vi "Main_verRockwell.vi"() -> ()   [LabVIEW 2014]
uses:
  <vilib>/ethernetip/ethernetip.llb/EthernetIP Tag Write BOOL.vi
  <vilib>/ethernetip/ethernetip.llb/EthernetIP Tag Write REAL.vi
  <vilib>/ethernetip/ethernetip.lvlib
  <vilib>/vision/driver/NI_Vision_Acquisition_Software.lvlib
panel:
  out "B":bool caption="Running"
  out "G":bool caption="Running"
  out "R":bool caption="Running"
  in  "Motion Speed":u32[](array[knob])=[80] scale=0.0..500.0
  in  "Linear Actuator Limit":u32(slide)=70 scale=0.0..100.0
  out "Linear Actuator Position Graph":dbl[][](graph)
  in  "Next Motion Delay":u32(slide)=200 scale=0.0..900.0
  in  "R Position":u32[](array[knob])=[35] scale=0.0..100.0
  in  "L Position":u32[](array[knob])=[40] scale=0.0..100.0
  in  "PORT":u16=50
  in  "IP":string="127.0.0.1"
  in  "Running Game":string="DiRT 3"
  out "Loop Count":i32=6322
  in  "Error RESET":bool
  in  "Simtools ON":bool
  in  "Motor Start":bool
  in  "Motor Reset":bool
  in  "STOP":bool
  in  "LED":bool
  in  "Axis":bool
  out "Running":bool
  in  "Error In":errorcluster
  out "Error Out":errorcluster
  out "R Position":dbl
  out "L Position":dbl
  out "Axis":string="L127R127C127"
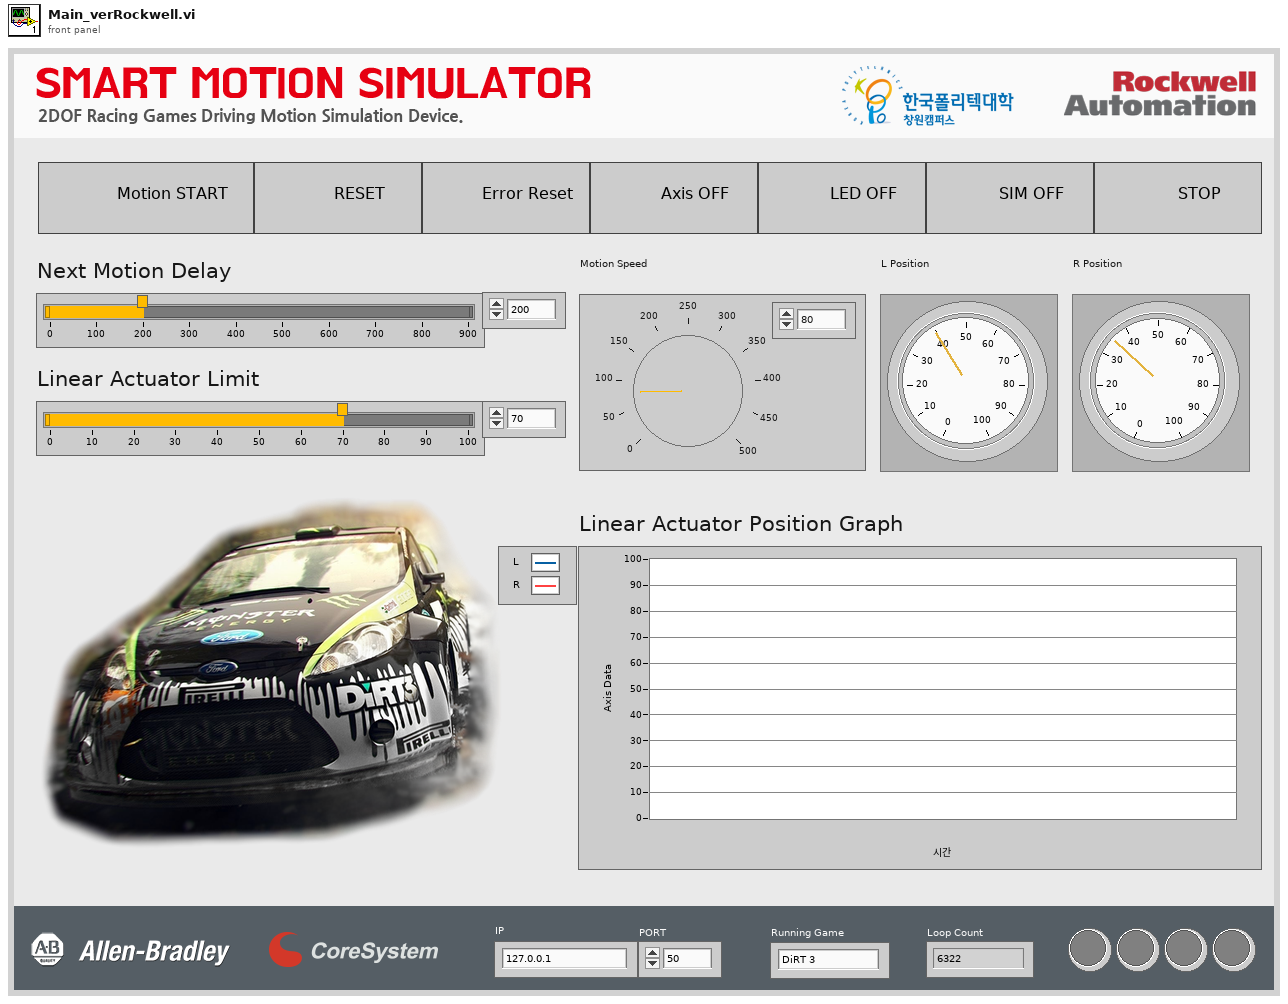
[diagram p1: front panel]
types:
  T1 = typedef "IMAQdx.ctl" = refnum<k21>
  T2 = typedef "IMAQ Image.ctl" = refnum<image>
  T3 = typedef "ethernetip.lvlib/ethernetip.ctl" = refnum<k21>
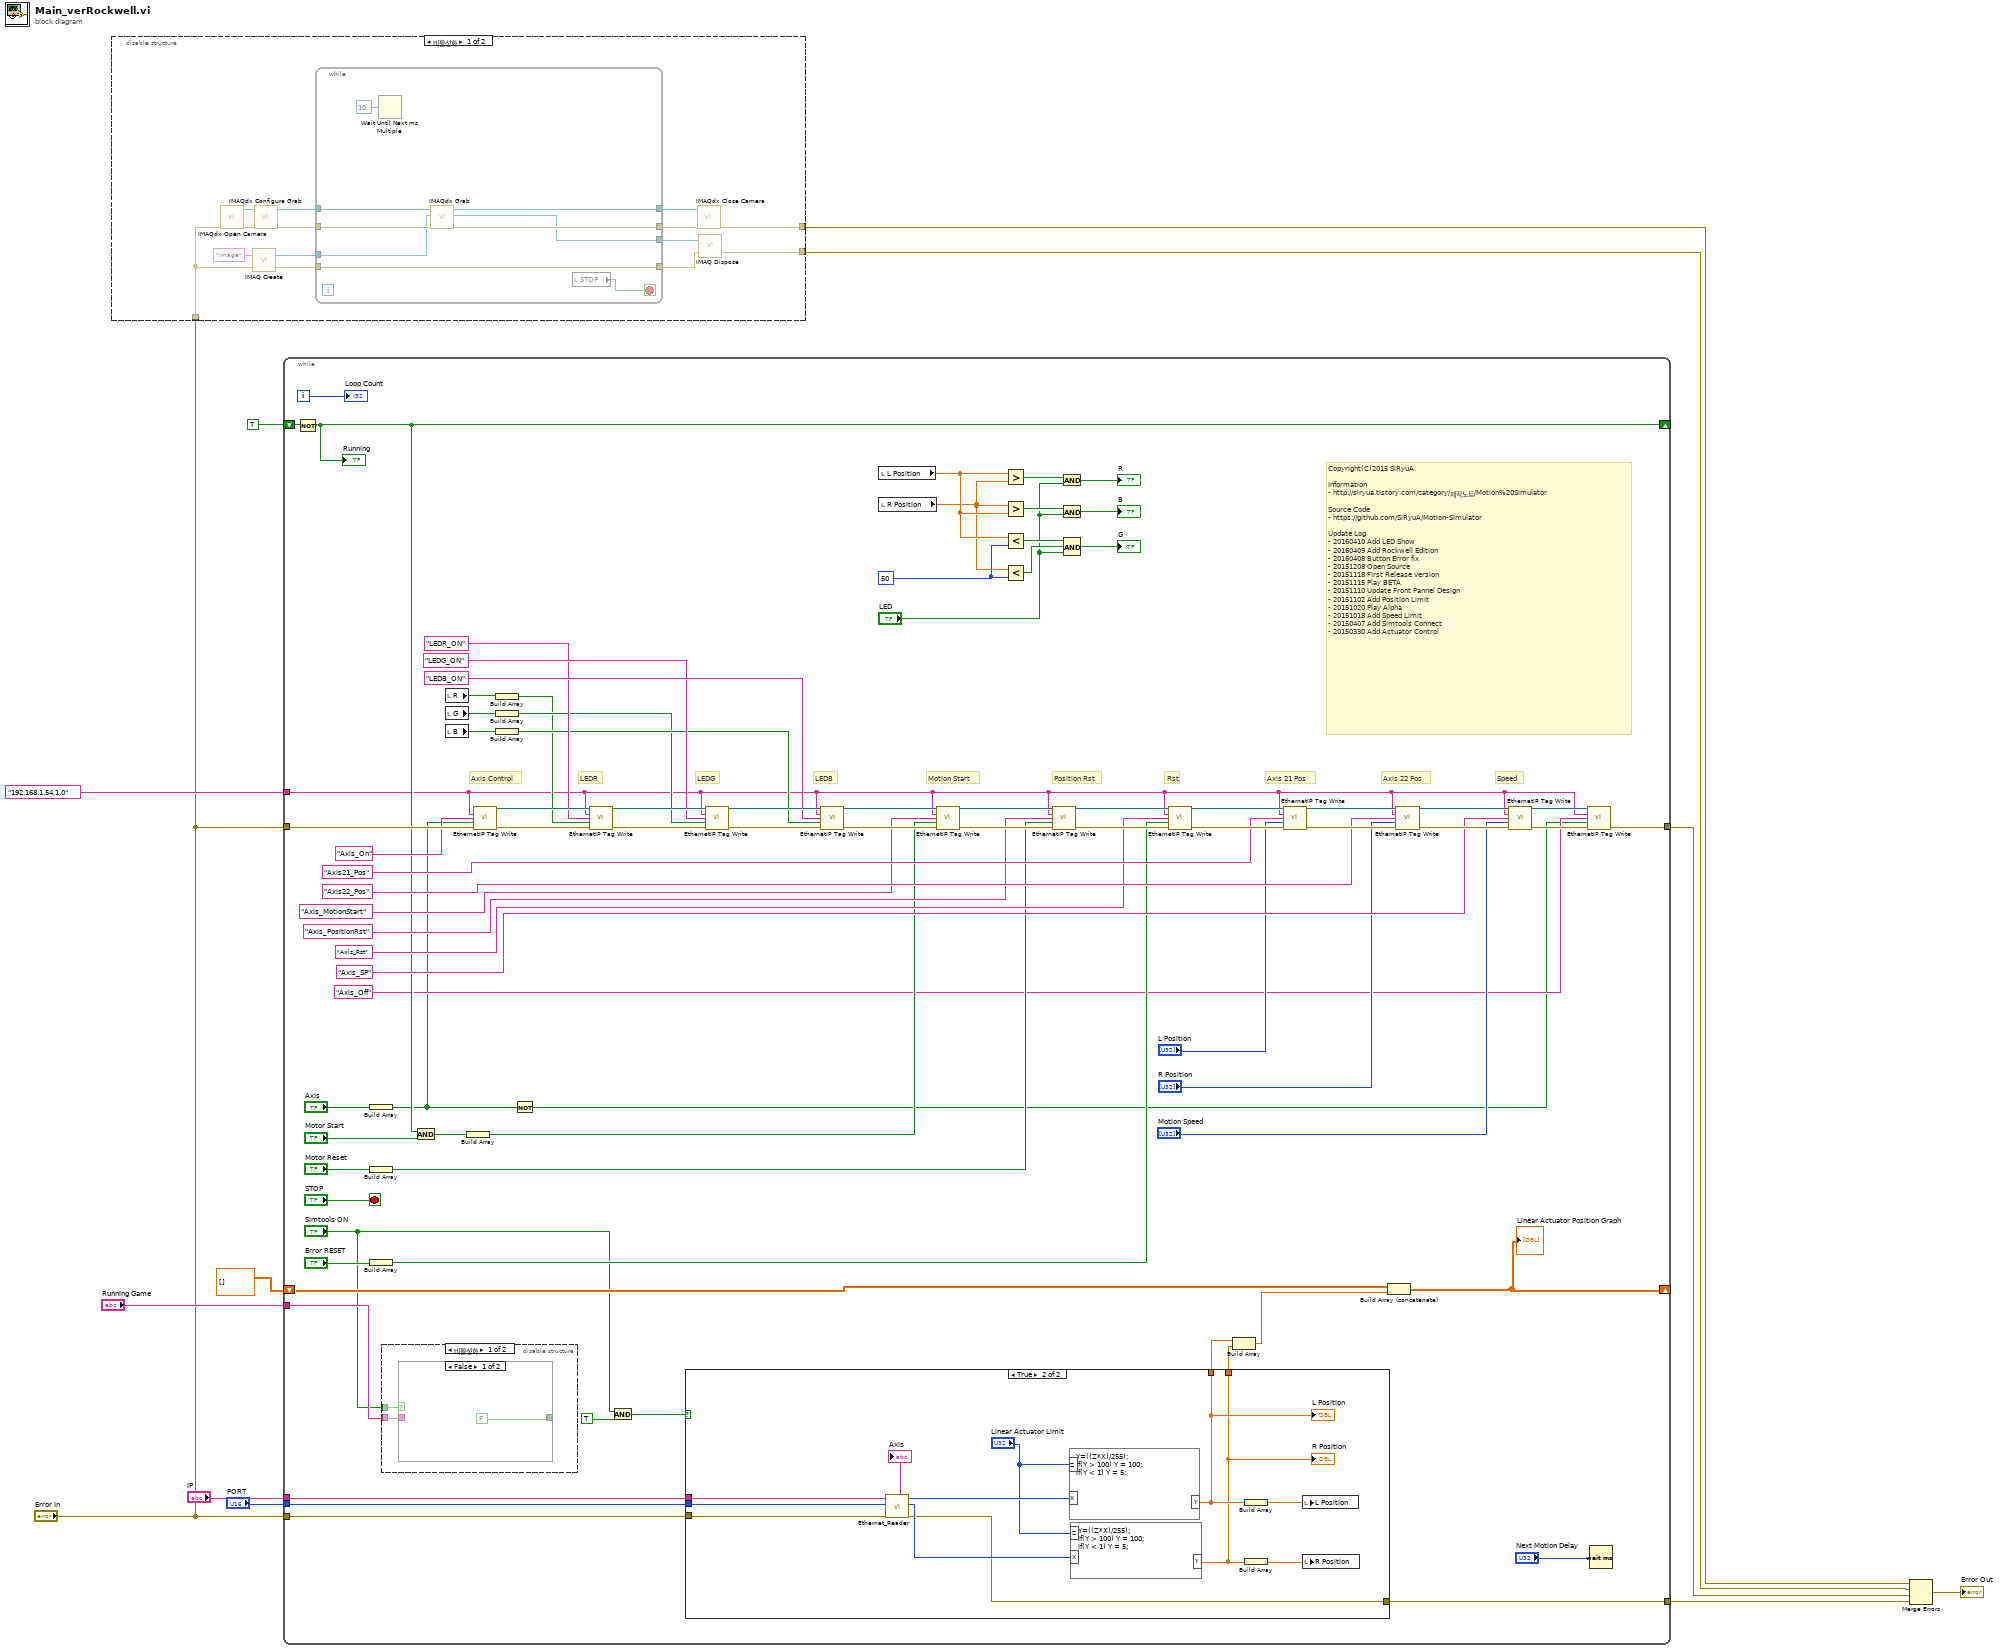
[diagram p0: block diagram]
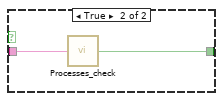
[diagram p3: hidden frame]
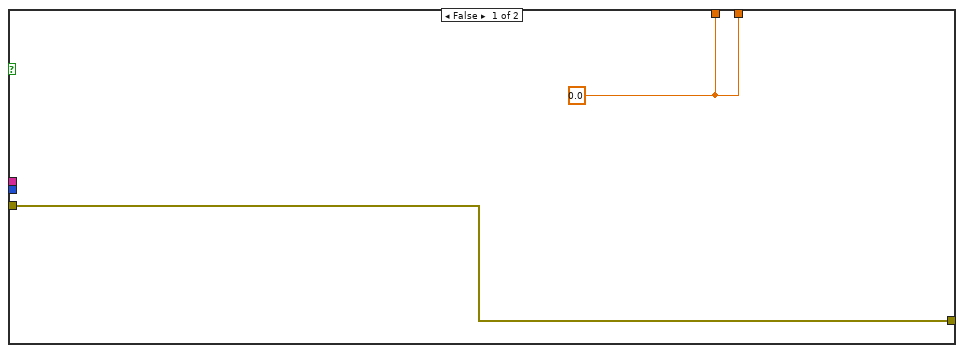
[diagram p5: hidden frame]
diagram:
  n1 = disable-structure shown="비활성화" {
    disable-tunnel: [w23 _] -> w6
    disable-tunnel: [w22 _] -> w5
    disable-tunnel: "Error In" -> [w21 _]
    frame Disabled {
      n2 = call <vilib>:"IMAQdx Open Camera.vi"("error in"=w21) -> ("error out"=w25:errorcluster, "Session Out"=w26:T1, "Session In"=w27:T1)  [unwired: 8 in]
      n3 = call "IMAQ Create"("Image Name"="Image", "error in (no error)"=w21) -> ("New Image"=w16:T2, "error out"=w14:errorcluster)  [unwired: 3 in]
      n4 = call <vilib>:"IMAQdx Configure Grab.vi"("error in"=w25, "Session In"=w26) -> ("error out"=w20:errorcluster, "Session Out"=w18:T1)  [unwired: 8 in]
      n5 = while {
        tunnel: w20 -> [w36]
        tunnel: [w35] -> w19
        tunnel: w18 -> [w34]
        tunnel: [w33] -> w17
        tunnel: w16 -> [w32]
        tunnel: [w31] -> w15
        tunnel: w14 -> [w31]
        tunnel: [w30] -> w13
        stop <- w29 stop-if-true
        n6 = Wait Until Next ms Multiple(millisecond multiple=u32 10 ("ms 배수")) -> ()  [unwired: 1 out]
        n7 = call <vilib>:"IMAQdx Grab.vi"("error in"=w36, "Image In"=w32, "Session In"=w34) -> ("error out"=w35:errorcluster, "Image Out"=w30:T2, "Session Out"=w33:T1)  [unwired: 5 in, 1 out]
        n8 = local read "STOP"() -> (w29:bool)
      }
      n9 = call <vilib>:"IMAQdx Close Camera.vi"("error in"=w19, "Session In"=w17) -> ("error out"=w22:errorcluster)  [unwired: 9 in]
      n10 = call "IMAQ Dispose"("Image"=w13, "error in (no error)"=w15) -> ("error out"=w23:errorcluster)  [unwired: 4 in]
    }
    frame Enabled {
    }
  }
  n11 = while {
    tunnel: "Error In" -> [w118]
    tunnel: [w41] -> w7
    tunnel: "192.168.1.54,1,0" ("Network Path") -> [w42]
    shift-right: [w67] -> _
    shift-left: TRUE -> [w68]
    tunnel: "Running Game" -> [w77]
    tunnel: "PORT" -> [w81]
    tunnel: "IP" -> [w80]
    tunnel: "Error In" -> [w79]
    tunnel: [w78] -> w2
    shift-right: [w72] -> _
    shift-left: dbl[][] [] -> [w75]
    i -> [w83]
    stop <- "STOP" stop-if-true
    w63 = 50
    # "Copyright(C)2015 SiRyuA.\n\nInformation\n- http://siryua.tistory.com/category/제작노트/Motion%20Simulator\n\nSource Code\n- https://github.com/SiRyuA/Motion-Simulator\n\nUpdate Log\n- 20160410 Add LED Show\n- 20160409 Add Rockwell Edition\n- 20160408 Button Error fix\n- 20151208 Open Source\n- 20151118 First Release version\n- 20151115 Play BETA\n- 20151110 Update Front Pannel Design\n- 20151102 Add Position Limit\n- 20151020 Play Alpha\n- 20151018 Add Speed Limit\n- 20150407 Add Simtools Connect\n- 20150330 Add Actuator Control"
    # "Speed"
    # "Rst"
    # "Position Rst"
    # "Motion Start"
    # "Axis 22 Pos"
    # "LEDB"
    # "LEDG"
    # "Axis 21 Pos"
    # "LEDR"
    # "Axis Control"
    n12 = Not(x=w68) -> (.not. x?=w67:bool)
    "Running" <- w67
    n13 = Build Array("Axis") -> (w38:bool[])
    n14 = Build Array("Motor Reset") -> (w86:bool[])
    n15 = Build Array("Error RESET") -> (w84:bool[])
    n16 = disable-structure shown="비활성화" {
      disable-tunnel: w77 -> [w120 _]
      disable-tunnel: "Simtools ON" -> [w119 _]
      frame Disabled {
        n17 = case shown="False" w119 {
          tunnel: w120 -> [_ w123]
          tunnel: [FALSE w122] -> _
          frame False {
          }
          frame True {
            n18 = call "Processes_check.vi"("검색 내용"=w123) -> ("불리언"=w122:bool)
          }
        }
      }
      frame Enabled {
      }
    }
    n19 = And(x=w67, y="Motor Start") -> (x .and. y?=w89:bool)
    n20 = local read "G"() -> (w48:bool)
    n21 = local read "R"() -> (w49:bool)
    n22 = local read "B"() -> (w47:bool)
    n23 = Build Array(w89) -> (w88:bool[])
    n24 = call-poly <vilib>:"EthernetIP Tag Write.vi"("Network Path"=w42, "Tag Name"="Axis_On", "Data"=w38, "error in"=w118) -> ("Session out"=w108:T3, "error out"=w117:errorcluster)  [unwired: 10 in]
    n25 = Build Array(w49) -> (w44:bool[])
    n26 = Build Array(w48) -> (w45:bool[])
    n27 = Build Array(w47) -> (w46:bool[])
    n28 = Not(x=w38) -> (.not. x?=w37:bool[])
    n29 = call-poly <vilib>:"EthernetIP Tag Write.vi"("Session in"=w108, "Network Path"=w42, "Tag Name"="LEDR_ON", "Data"=w44, "error in"=w117) -> ("Session out"=w107:T3, "error out"=w116:errorcluster)  [unwired: 9 in]
    n30 = And(x="Simtools ON", y=TRUE) -> (x .and. y?=w82:bool)
    n31 = case shown="True" w82 {
      tunnel: w81 -> [_ w134]
      tunnel: w80 -> [_ w133]
      tunnel: w79 -> [w125 w130]
      tunnel: [w125 w129] -> w78
      tunnel: [w124 w127] -> w70
      tunnel: [w124 w126] -> w69
      frame False {
        w124 = 0.0
      }
      frame True {
        n32 = call "Ethernet_Reader.vi"("에러 입력(에러 없음)"=w130, "포트"=w134, "IP"=w133) -> ("에러 출력"=w129:errorcluster, "R"=w135:u32, "L"=w136:u32, "Axis"=→"Axis":string)  [unwired: 5 in]
        n33 = formula code="Y=((Z*X)/255);\nif(Y > 100) Y = 100;\nif(Y < 1) Y = 5;"("X"=w136, "Z"="Linear Actuator Limit") -> ("Y"=w127:dbl)
        "L Position" <- w127
        n34 = formula code="Y=((Z*X)/255);\nif(Y > 100) Y = 100;\nif(Y < 1) Y = 5;"("X"=w135, "Z"="Linear Actuator Limit") -> ("Y"=w126:dbl)
        "R Position" <- w126
        n35 = Build Array(w127) -> (w132:dbl[])
        n36 = Build Array(w126) -> (w131:dbl[])
        n37 = local write "L Position"(w132) -> ()
        n38 = local write "R Position"(w131) -> ()
      }
    }
    n39 = call-poly <vilib>:"EthernetIP Tag Write.vi"("Session in"=w107, "Network Path"=w42, "Tag Name"="LEDG_ON", "Data"=w45, "error in"=w116) -> ("Session out"=w106:T3, "error out"=w115:errorcluster)  [unwired: 9 in]
    n40 = call-poly <vilib>:"EthernetIP Tag Write.vi"("Session in"=w106, "Network Path"=w42, "Tag Name"="LEDB_ON", "Data"=w46, "error in"=w115) -> ("Session out"=w105:T3, "error out"=w114:errorcluster)  [unwired: 9 in]
    n41 = local read "L Position"() -> (w54:dbl)
    n42 = local read "R Position"() -> (w53:dbl)
    n43 = call-poly <vilib>:"EthernetIP Tag Write.vi"("Session in"=w105, "Network Path"=w42, "Tag Name"="Axis_MotionStart", "Data"=w88, "error in"=w114) -> ("Session out"=w104:T3, "error out"=w113:errorcluster)  [unwired: 9 in]
    n44 = Greater?(x=w54, y=w53) -> (0:w62:bool)
    n45 = Greater?(x=w53, y=w54) -> (0:w61:bool)
    n46 = Less?(x=w54, y=w63) -> (x < y?=w60:bool)
    n47 = Less?(x=w53, y=w63) -> (x < y?=w59:bool)
    n48 = call-poly <vilib>:"EthernetIP Tag Write.vi"("Session in"=w104, "Network Path"=w42, "Tag Name"="Axis_PositionRst", "Data"=w86, "error in"=w113) -> ("Session out"=w103:T3, "error out"=w112:errorcluster)  [unwired: 9 in]
    n49 = And(x=w62, y="LED") -> (x .and. y?=→"R":bool)
    n50 = And(x=w61, y="LED") -> (x .and. y?=→"B":bool)
    n51 = Compound Arithmetic op=AND(w60, w59, "LED") -> (→"G":bool)
    n52 = call-poly <vilib>:"EthernetIP Tag Write.vi"("Session in"=w103, "Network Path"=w42, "Tag Name"="Axis_Rst", "Data"=w84, "error in"=w112) -> ("Session out"=w102:T3, "error out"=w111:errorcluster)  [unwired: 9 in]
    n53 = Build Array(w70, w69) -> (w71:dbl[])
    n54 = call-poly <vilib>:"EthernetIP Tag Write.vi"("Session in"=w102, "Network Path"=w42, "Tag Name"="Axis21_Pos", "Data"="L Position", "error in"=w111) -> ("Session out"=w101:T3, "error out"=w110:errorcluster)  [unwired: 9 in]
    n55 = Build Array (concatenate)(w75, w71) -> (w72:dbl[][])
    "Linear Actuator Position Graph" <- w72
    n56 = call-poly <vilib>:"EthernetIP Tag Write.vi"("Session in"=w101, "Network Path"=w42, "Tag Name"="Axis22_Pos", "Data"="R Position", "error in"=w110) -> ("Session out"=w100:T3, "error out"=w109:errorcluster)  [unwired: 9 in]
    n57 = call-poly <vilib>:"EthernetIP Tag Write.vi"("Session in"=w100, "Network Path"=w42, "Tag Name"="Axis_SP", "Data"="Motion Speed", "error in"=w109) -> ("Session out"=w43:T3, "error out"=w40:errorcluster)  [unwired: 9 in]
    n58 = call-poly <vilib>:"EthernetIP Tag Write.vi"("Session in"=w43, "Network Path"=w42, "Tag Name"="Axis_Off", "Data"=w37, "error in"=w40) -> ("error out"=w41:errorcluster)  [unwired: 9 in, 1 out]
    n59 = Wait (ms)(milliseconds to wait="Next Motion Delay") -> ()  [unwired: 1 out]
    "Loop Count" <- w83
  }
  n60 = Merge Errors(w5, w6, w7, w2) -> (→"Error Out":errorcluster)
